vi "iterate-types.vi"() -> ()   [LabVIEW 2020]
uses:
  G-Embedded-Python-Interpreter-Toolkit/G-Embedded-Python-Interpreter-Toolkit.lvlib
  <vilib>/Utility/Data Type/NI_Data Type.lvlib
  <vilib>/Utility/Data Type/Type Definitions/Data Type.ctl
panel:
  out "type":T1
  out "number of dimensions":i32
  out "Name":string
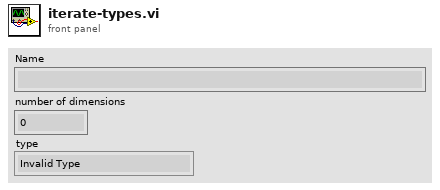
[diagram p1: front panel]
types:
  T1 = typedef "NI_Data Type.lvlib/Data Type.ctl" = enum8{"Invalid Type", "Void", "I8", "I16", "I32", "I64", "U8", "U16", "U32", "U64", "Single Float", "Double Float", "Extended Float", "Single Complex", "Double Complex", "Extended Complex", "Enum U8", "Enum U16", "Enum U32", "Enum U64", "Single Float With Unit", "Double Float With Unit", "Extended Float With Unit", "Single Complex with Unit", "Double Complex with Unit", "Extended Complex with Unit", "Boolean", "String", "Path", "Picture", "Tag", "Array", "Cluster", "Variant", "LV Variant", "Waveform", "Timestamp", "Digital Waveform", "Digital Data", "ExpressData", "Refnum", "External Data", "VI", "Poly VI", "LabVIEW Class Instance", "Fixed Point", "Set Collection", "Map Collection"}
  T2 = typedef "G-Embedded-Python-Interpreter-Toolkit.lvlib/Python Object Reference.ctl" = refnum<k1>
  T3 = cluster{"Null Python Object Refnum":T2, i32[], void}
  T4 = typedef "NI_Data Type.lvlib/Type Definition Info.ctl" = cluster{"Name":string, "Timestamp":u32}
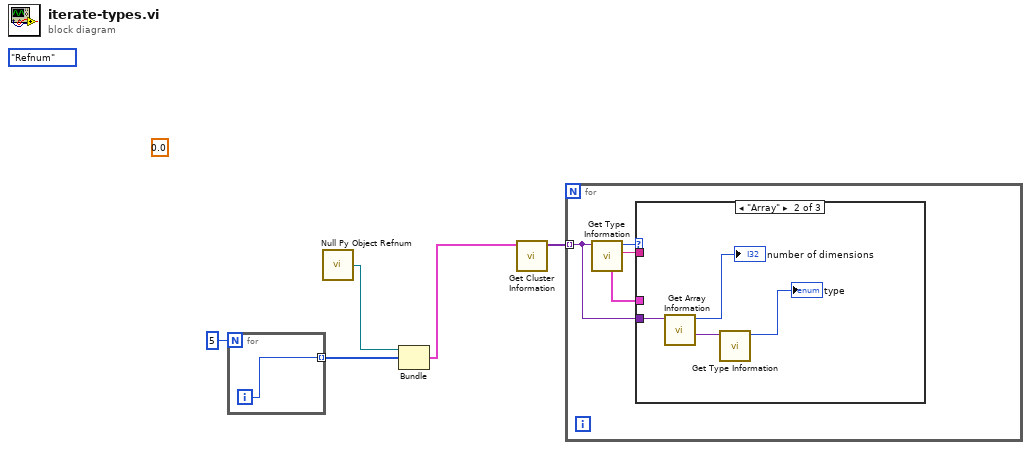
[diagram p0: block diagram]
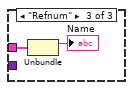
[diagram p3: hidden frame]
diagram:
  (unwired) 0.0
  (unwired) Data_Type."Refnum" ("type")
  n1 = for {
    N: 5 -> [_]
    tunnel: [w6] -> w5 mode=indexing
    i -> [w6]
  }
  n2 = call "Null Py Object Refnum.vi"() -> ("Null Python Object Refnum"=w3:T2)
  n3 = Bundle("Null Python Object Refnum"=w3, w5) -> (w2:T3)  [unwired: 2 in]
  n4 = call <vilib>:"Get Cluster Information.vi"("variant"=w2) -> ("cluster elements"=w1:variant[])  [unwired: 9 in, 1 out]
  n5 = for {
    tunnel: w1 -> [w7] mode=indexing
    n6 = call <vilib>:"Get Type Information.vi"("variant"=w7) -> ("name"=w8:string, "type"=w9:T1, "type definition info"=w10:T4)  [unwired: 6 in, 2 out]
    n7 = case shown="\"Array\"" w9 {
      tunnel: w10 -> [_ _ w16]
      tunnel: w8 -> [_ _ _]
      tunnel: w7 -> [_ w14 _]
      frame Default {
      }
      frame "Array" {
        n8 = call <vilib>:"Get Array Information.vi"("variant"=w14) -> ("array element data type"=w13:variant, "number of dimensions"=→"number of dimensions":i32)  [unwired: 7 in, 2 out]
        n9 = call <vilib>:"Get Type Information.vi"("variant"=w13) -> ("type"=→"type":T1)  [unwired: 6 in, 4 out]
      }
      frame "Refnum" {
        n10 = Unbundle(w16) -> ("Name"=→"Name":string)  [unwired: 1 out]
      }
    }
  }
